vi "Periodic Tasks.vi"(8 "error in":errorcluster) -> ()   [LabVIEW 2016]
doc: "This VI runs in parallel to other tasks. It can contain as many user-defined periodic loops as you need. These can carry out PID or other sorts of timed response."
uses:
  Robot Global Data.vi
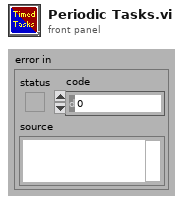
[diagram p1: front panel]
types:
  T1 = typedef "WPI_EncoderDevRef.ctl" = cluster{"DevStatus":errorcluster, "EncoderIndex":T2, "CounterIndex":T3, "DistancePerCount":dbl, "Decoding Type":T4}
  T2 = typedef "FPGA_EncoderIdx.ctl" = enum8{"Enc 0", "Enc 1", "Enc 2", "Enc 3", "Enc 4", "Enc 5", "Enc 6", "Enc 7", "Invalid"}
  T3 = typedef "FPGA_CounterCtrSystemIndex.ctl" = enum8{"Ctr 0", "Ctr 1", "Ctr 2", "Ctr 3", "Ctr 4", "Ctr 5", "Ctr 6", "Ctr 7", "Invalid"}
  T4 = typedef "WPI_EncoderType.ctl" = enum16{"1x", "2x", "4x"}
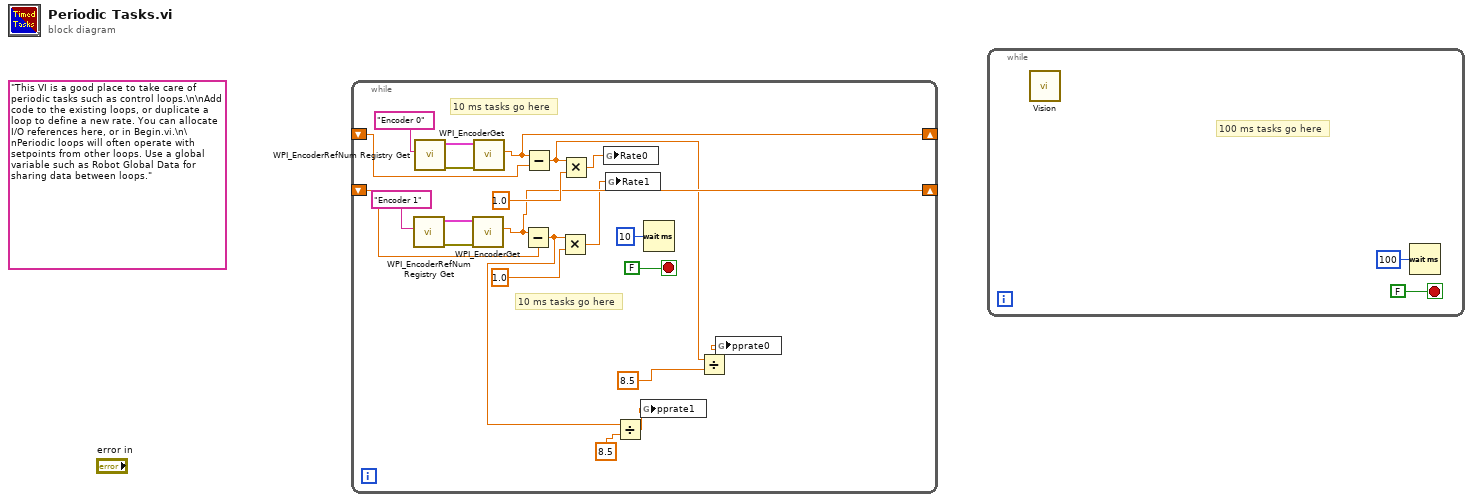
[diagram p0: block diagram]
diagram:
  (unwired) "This VI is a good place to take care of periodic tasks such as control loops.\n\nAdd code to the existing loops, or duplicate a loop to define a new rate. You can allocate I/O references here, or in Begin.vi.\n\nPeriodic loops will often operate with setpoints from other loops. Use a global variable such as Robot Global Data for sharing data between loops."
  n1 = while {
    shift-right: [w17] -> _
    shift-left: _ -> [w16]
    shift-right: [w9] -> _
    shift-left: _ -> [w10]
    stop <- FALSE stop-if-true
    # "10 ms tasks go here"
    # "10 ms tasks go here"
    n2 = call <vilib>:"WPI_EncoderRefNum Registry Get.vi"("refnum name"="Encoder 1") -> ("error out"=w14:errorcluster, "EncoderDevRef"=w13:T1)  [unwired: 9 in]
    n3 = call <vilib>:"WPI_EncoderRefNum Registry Get.vi"("refnum name"="Encoder 0") -> ("error out"=w20:errorcluster, "EncoderDevRef"=w19:T1)  [unwired: 9 in]
    n4 = call <vilib>:"WPI_EncoderGet.vi"("error in (no error)"=w14, "EncoderDevRef"=w13) -> ("Distance"=w9:dbl)  [unwired: 4 in, 5 out]
    n5 = call <vilib>:"WPI_EncoderGet.vi"("error in (no error)"=w20, "EncoderDevRef"=w19) -> ("Distance"=w17:dbl)  [unwired: 4 in, 5 out]
    n6 = Subtract(x=w9, y=w10) -> (x-y=w1:dbl)
    n7 = Subtract(x=w17, y=w16) -> (x-y=w2:dbl)
    n8 = Multiply(x=w1, y=1.0) -> (x*y=w7:dbl)
    n9 = Multiply(x=w2, y=1.0) -> (x*y=w8:dbl)
    n10 = global write "Robot Global Data.vi" "Rate0"(w8) -> ()
    n11 = global write "Robot Global Data.vi" "Rate1"(w7) -> ()
    n12 = Divide(x=w1, y=8.5) -> (x/y=w6:dbl)
    n13 = global write "Robot Global Data.vi" "pprate1"(w6) -> ()
    n14 = Wait (ms)(milliseconds to wait=u32 10) -> ()  [unwired: 1 out]
    n15 = Divide(x=w2, y=8.5) -> (x/y=w5:dbl)
    n16 = global write "Robot Global Data.vi" "pprate0"(w5) -> ()
  }
  n17 = while {
    stop <- FALSE stop-if-true
    # "100 ms tasks go here"
    n18 = call "Vision.vi"() -> ()  [unwired: 12 in]
    n19 = Wait (ms)(milliseconds to wait=u32 100) -> ()  [unwired: 1 out]
  }
